vi "ABR-Save Data.vi"(0 "raw data filestem":path, 1 "State (in)":T7, 5 "Params":T1={"CAP or ABR"=enum."ABR", "Stimulus"={"Ear"=enum."Left", "Start (dB)"=0, "Waveform"=enum."TONE PIP", "Stop (dB)"=30, "Frequency (kHz)"=16.0, "Step (dB)"=5, "Rep rate (/sec)"=30.0, "Alternate Polarity"=FALSE}, "Response"={"Gain"=10000, "Averages"=512, "Window (ms)"=8.5, "Thr Fast Steps"=8.5}, "Hidden"={"AI Samp Rate Hz"=25000.0, "AO Samp Rate Hz"=100000.0, "Duration (ms)"=5.0, "Ramp (ms)"=0.5, "Click width (us)"=0.0, "ITI"=enum."Rate", "Save raw"=FALSE}, "Version"=0} {"Response"."Thr Fast Steps" format="%.2f"; "Response"."Window (ms)" format="%.2f"; "Stimulus"."Frequency (kHz)" format="%.2f"; "Stimulus"."Start (dB)" step=5}, 9 "Aborted?":bool, 11 "error in (no error)":errorcluster, 12 "Analysis":T5, 13 "Notes":string) -> (3 "State (out)":T7, 4 "Run #":i16, 6 "Datafile path":path, 10 "Saved?":bool, 15 "error out":errorcluster)   [LabVIEW 2020]
uses:
  CFTS Main Panel SubVIs/CFTS-Experiment State.ctl
  TypeDefs/ABR-Analysis State.ctl
  Threshold Estimation VIs/ABR3-Threshold Estimation Result.ctl
  TypeDefs/ABR-Parameters.ctl
  TypeDefs/ABR-Stimulus.ctl
  TypeDefs/ABR-Response.ctl
  TypeDefs/ABR-Hidden Params.ctl
  epl-vi-lib/Utility VIs/File IO VIs/Configuration File Wrapper VIs/Config-Read Key (string).vi
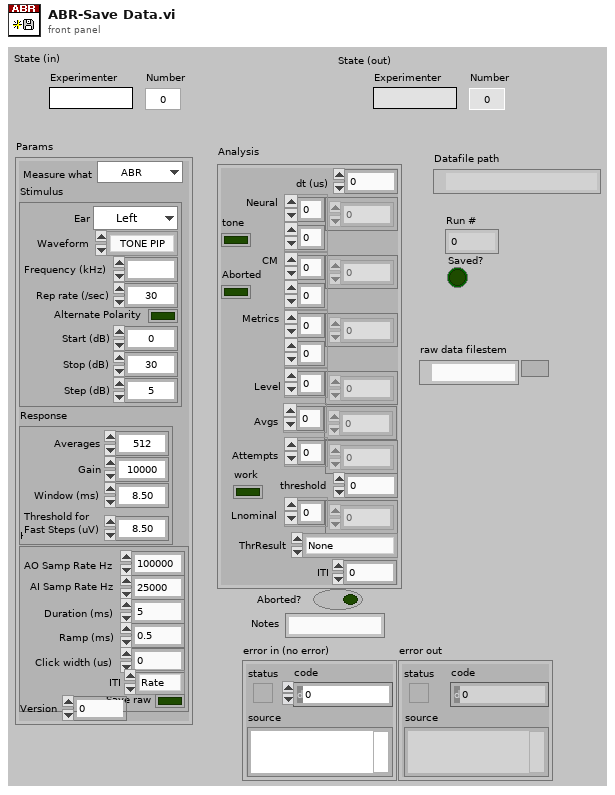
[diagram p1: front panel]
types:
  T1 = typedef "ABR-Parameters.ctl" = cluster{"CAP or ABR":enum16{"CAP", "ABR"}, "Stimulus":T2, "Response":T3, "Hidden":T4, "Version":i32}
  T2 = typedef "ABR-Stimulus.ctl" = cluster{"Ear":enum16{"Right", "Left", "Bone"}, "Start (dB)":i32, "Waveform":enum16{"TONE PIP", "CLICK"}, "Stop (dB)":i32, "Frequency (kHz)":ext, "Step (dB)":i32, "Rep rate (/sec)":dbl, "Alternate Polarity":bool}
  T3 = typedef "ABR-Response.ctl" = cluster{"Gain":i32, "Averages":i32, "Window (ms)":sgl, "Thr Fast Steps":sgl}
  T4 = typedef "ABR-Hidden Params.ctl" = cluster{"AI Samp Rate Hz":dbl, "AO Samp Rate Hz":dbl, "Duration (ms)":dbl, "Ramp (ms)":dbl, "Click width (us)":dbl, "ITI":enum16{"Rate", "Interval"}, "Save raw":bool}
  T5 = typedef "ABR-Analysis State.ctl" = cluster{"dt (us)":dbl, "Neural":dbl[][], "CM":dbl[][], "Metrics":dbl[][], "Level":dbl[], "Avgs":i32[], "Attempts":i32[], "Aborted":bool, "threshold":dbl, "Lnominal":dbl[], "tone":bool, "work":bool, "ThrResult":T6, "ITI":dbl}
  T6 = typedef "ABR3-Threshold Estimation Result.ctl" = enum16{"None", "Power", "Sigmoid", "Power (noisy)", "Suprathreshold", "Invalid"}
  T7 = typedef "CFTS-Experiment State.ctl" = cluster{"Experimenter":string, "Number":u32, "Right":string, "Left":string, "Data Folder":path, "State File":path, "Version Info":string, "End Exposure Time":dbl, "Exposure Duration":string, "Run #":cluster{"CAP":i16, "ABR":i16, "DP":i16, "VsEP":i16, "MeasSeq":i16, "SubSeq":i16, "SFOAE":i16}}
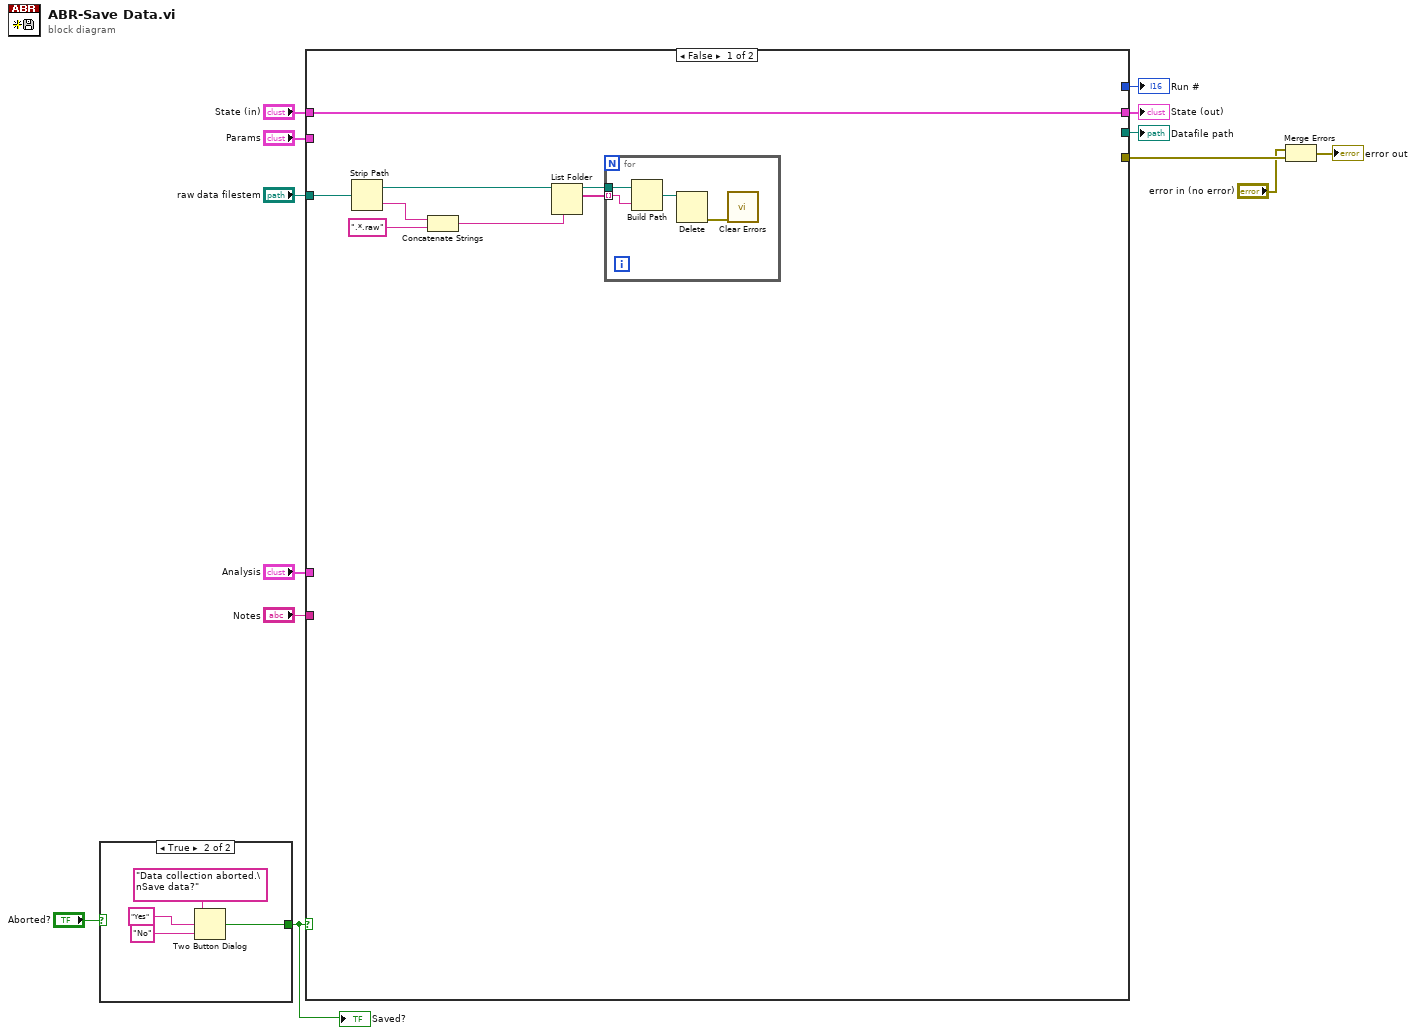
[diagram p0: block diagram]
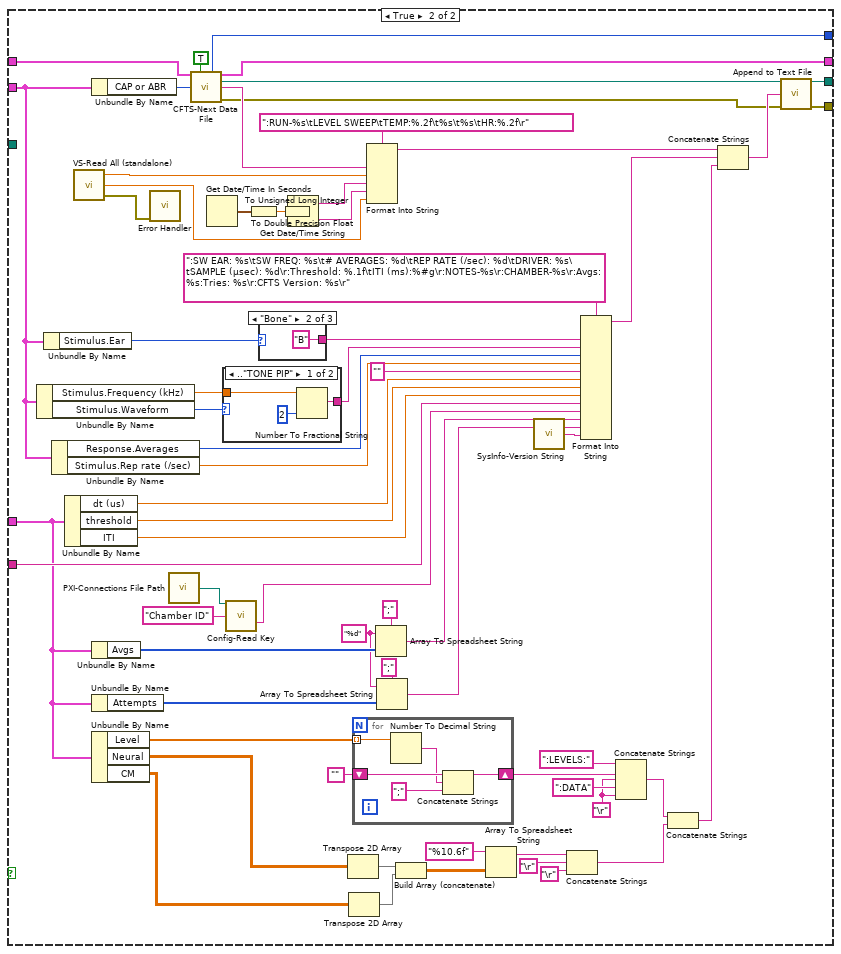
[diagram p2: hidden frame]
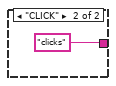
[diagram p3: hidden frame]
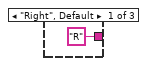
[diagram p4: hidden frame]
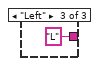
[diagram p5: hidden frame]
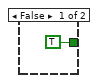
[diagram p6: hidden frame]
diagram:
  n1 = case shown="True" "Aborted?" {
    tunnel: [TRUE ("T button?") w15] -> w3
    frame False {
    }
    frame True {
      n2 = Two Button Dialog(message="Data collection aborted.\nSave data?", 1:"No" ("F button name (\"Cancel\")"), 2:"Yes" ("T button name (\"OK\")")) -> (T button?=w15:bool)
    }
  }
  "Saved?" <- w3
  n3 = case shown="False" w3 {
    tunnel: "State (in)" -> [w26 w96]
    tunnel: [w26 w95] -> w12
    tunnel: [_ w82] -> w11
    tunnel: "Notes" -> [_ w73]
    tunnel: [_ w72] -> w8
    tunnel: "Analysis" -> [_ w36]
    tunnel: [_ w52] -> w6
    tunnel: "Params" -> [_ w37]
    tunnel: "raw data filestem" -> [w24 _]
    frame False {
      n4 = Strip Path(path=w24) -> (stripped path=w23:path, name=w22:string)
      n5 = Concatenate Strings(w22, ".*.raw" ("format string")) -> (w21:string)
      n6 = List Folder(path=w23, pattern=w21) -> (path out=w20:path, filenames=w19:string[])  [unwired: 2 in, 2 out]
      n7 = for {
        tunnel: w20 -> [w29]
        tunnel: w19 -> [w28] mode=indexing
        n8 = Build Path(base path=w29, name or relative path=w28) -> (appended path=w27:path)
        n9 = Delete(path (use dialog)=w27) -> (error out=w30:errorcluster)  [unwired: 4 in, 2 out]
        n10 = call <vilib>:"Clear Errors.vi"("error in (no error)"=w30) -> ()  [unwired: 5 in, 2 out]
      }
    }
    frame True {
      w42 = "%d" ("format string")
      w66 = "\r"
      n11 = Unbundle By Name(w37) -> ("Stimulus.Frequency (kHz)"=w55:ext, "Stimulus.Waveform"=w77:enum16{"TONE PIP", "CLICK"})
      n12 = Unbundle By Name(w37) -> ("Stimulus.Ear"=w80:enum16{"Right", "Left", "Bone"})
      n13 = Unbundle By Name(w37) -> ("Response.Averages"=w76:i32, "Stimulus.Rep rate (/sec)"=w75:dbl)
      n14 = Unbundle By Name(w36) -> ("dt (us)"=w35:dbl, "threshold"=w32:dbl, "ITI"=w31:dbl)
      n15 = call "VS-Read All (standalone).vi"() -> ("error out"=w50:errorcluster, "Heart Rate (bpm)"=w49:dbl, "Temperature (C)"=w51:dbl)  [unwired: 3 in]
      n16 = Unbundle By Name(w37) -> ("CAP or ABR"=w71:enum16{"CAP", "ABR"})
      n17 = Unbundle By Name(w36) -> ("Avgs"=w46:i32[])
      n18 = Unbundle By Name(w36) -> ("Attempts"=w44:i32[])
      n19 = Unbundle By Name(w36) -> ("Level"=w38:dbl[], "Neural"=w54:dbl[][], "CM"=w53:dbl[][])
      n20 = call "Error Handler.vi"("error in (no error)"=w50) -> ()  [unwired: 13 in, 2 out]
      n21 = call "PXI-Connections File Path.vi"() -> ("Path"=w34:path)  [unwired: 1 in]
      n22 = call "CFTS-Next Data File.vi"("Expt State"=w96, "Allow overwrite"=TRUE, "Data Type"=w71) -> ("Run #"=w72:i16, "Expt State out"=w95:T7, "Datafile path"=w85:path, "run #"=w88:string, "error out"=w83:errorcluster)  [unwired: 8 in]
      n23 = Get Date/Time In Seconds() -> (seconds since 1Jan1904=w92:timestamp)
      n24 = case shown="..\"TONE PIP\"" w77 {
        tunnel: [w98 "clicks"] -> w78
        tunnel: w55 -> [w99 _]
        frame .."TONE PIP" {
          n25 = Number To Fractional String(number=w99, precision (6)=2) -> (F-format string=w98:string)  [unwired: 2 in]
        }
        frame "CLICK" {
        }
      }
      n26 = call-poly "Config-Read Key.vi"("configuration file path"=w34, "key"="Chamber ID" ("string")) -> ("value"=w33:string)  [unwired: 10 in, 3 out]
      n27 = To Double Precision Float(number=w92) -> (double precision float=w91:dbl)
      n28 = case shown="\"Bone\"" w80 {
        tunnel: ["R" "B" "L"] -> w79
        frame "Right", Default {
        }
        frame "Bone" {
        }
        frame "Left" {
        }
      }
      n29 = To Unsigned Long Integer(number=w91) -> (unsigned 32bit integer=w90:u32)
      n30 = Get Date/Time String(seconds (now)=w90) -> (date string=w93:string, time string=w94:string)  [unwired: 2 in]
      n31 = Transpose 2D Array(2D array=w54) -> (transposed array=w60:dbl[][])
      n32 = Transpose 2D Array(2D array=w53) -> (transposed array=w59:dbl[][])
      n33 = for {
        shift-right: [w105] -> w67
        shift-left: "" -> [w108]
        tunnel: w38 -> [w104] mode=indexing
        n34 = Number To Decimal String(number=w104) -> (decimal integer string=w107:string)  [unwired: 1 in]
        n35 = Concatenate Strings(w108, w107, ";") -> (w105:string)
      }
      n36 = Format Into String(format string=":RUN-%s\tLEVEL SWEEP\tTEMP:%.2f\t%s\t%s\tHR:%.2f\r", w88, w51, w93, w94, w49) -> (resulting string=w87:string)  [unwired: 2 in, 1 out]
      n37 = Array To Spreadsheet String(delimiter (Tab)=";", array=w46, 3:w42) -> (spreadsheet string=w45:string)
      n38 = Array To Spreadsheet String(delimiter (Tab)=";", array=w44, 3:w42) -> (spreadsheet string=w41:string)
      n39 = Build Array (concatenate)(w60, w59) -> (w58:dbl[][])
      n40 = Array To Spreadsheet String(array=w58, 3:"%10.6f") -> (spreadsheet string=w63:string)  [unwired: 1 in]
      n41 = call "SysInfo-Version String.vi"() -> ("Version String"=w40:string)  [unwired: 1 in]
      n42 = Concatenate Strings(w63, "\r", "\r") -> (w57:string)
      n43 = Format Into String(format string=":SW EAR: %s\tSW FREQ: %s\t# AVERAGES: %d\tREP RATE (/sec): %d\tDRIVER: %s\tSAMPLE (µsec): %d\r:Threshold: %.1f\tITI (ms):%#g\r:NOTES-%s\r:CHAMBER-%s\r:Avgs: %s:Tries: %s\r:CFTS Version: %s\r", w79, w78, w76, w75, "" ("input 5"), w35, w32, w31, w73, w33, w45, w41, w40) -> (resulting string=w81:string)  [unwired: 2 in, 1 out]
      n44 = Concatenate Strings(":LEVELS:", w67, w66, ":DATA", w66) -> (w65:string)
      n45 = Concatenate Strings(w65, w57) -> (w56:string)
      n46 = Concatenate Strings(w87, w81, w56) -> (w84:string)
      n47 = call "Append to Text File.vi"("file path"=w85, "text"=w84, "error in (no error)"=w83) -> ("file path out"=w82:path, "error out"=w52:errorcluster)  [unwired: 11 in]
    }
  }
  "State (out)" <- w12
  "Datafile path" <- w11
  "Run #" <- w8
  n48 = Merge Errors("error in (no error)", w6) -> (→"error out":errorcluster)
